vi "lockin - zero amplitude.vi"(6 "measure\noffset?":bool, 8 "error in (no error)":errorcluster, 11 "Lockin":refnum<class "Instrument.Lockin.lvclass">) -> (0 "error out":errorcluster, 3 "Lockin out":refnum<class "Instrument.Lockin.lvclass">)   [LabVIEW 2016, in "Instrument.Lockin.lvclass"]
uses:
  Instrument.Lockin.lvclass
  Instrument.Lockin.lvclass/Instrument.Lockin.ctl
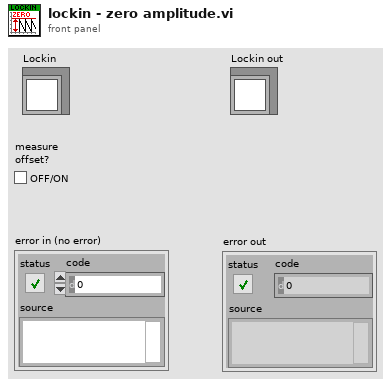
[diagram p1: front panel]
types:
  T1 = typedef "Instrument.Lockin.lvclass/AO_Amp-array.ctl" = dbl[]
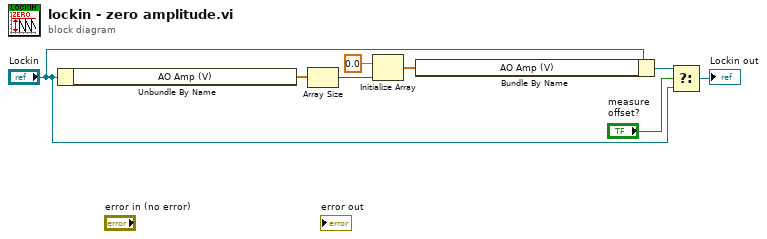
[diagram p0: block diagram]
diagram:
  n1 = Unbundle By Name("Lockin") -> ("AO Amp (V)"=w6:T1)
  n2 = Array Size(array=w6) -> (size(s)=w5:i32)
  n3 = Initialize Array(0.0 ("element"), w5) -> (w8:dbl[])
  n4 = Bundle By Name(cluster="Lockin", "AO Amp (V)"=w8) -> (w4:refnum<class "Instrument.Lockin.lvclass">)
  n5 = Select(t=w4, s="measure\noffset?", f="Lockin") -> (s? t:f=→"Lockin out":refnum<class "Instrument.Lockin.lvclass">)
